vi "Constants.vi"() -> ()   [LabVIEW 2017, in "Exercise 7.1 Shared.lvlib"]
doc: "Use this Global VI to access the GUIDs assigned to the page resources of the Custom Device."
uses:
  Exercise 7.1 Shared.lvlib
panel:
  in  "Tab Control":enum32{"GUIDS", "Constants", "Properties"}(tab)
  in  "Exercise 7.1":string="365fcfbc-9e44-44c7-b391-d2378ce24c16"
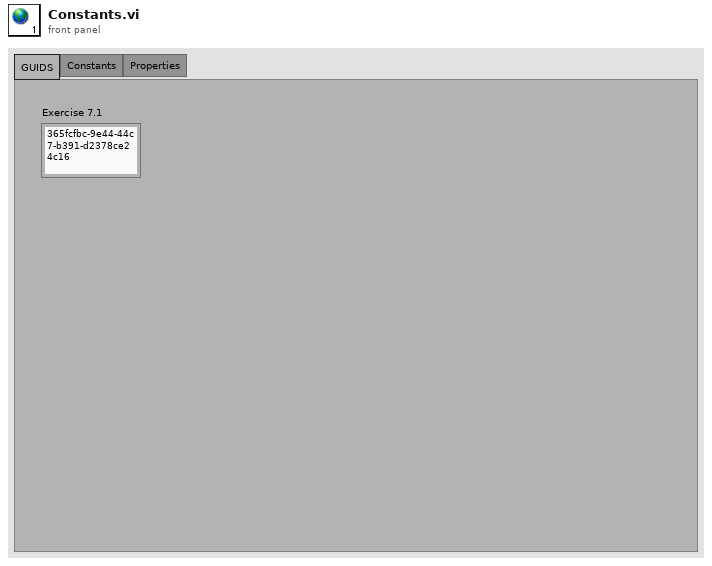
[diagram p1: front panel]
diagram:
